vi "Stop Core.vi"(10 "final error code":i32, 11 "WT1600 in":refnum<class "WT1600.lvclass">) -> (3 "WT1600 out":refnum<class "WT1600.lvclass">)   [LabVIEW 2013, in "Universal Power Meter.lvlib" / "WT1600.lvlib" / "WT1600.lvclass"]
doc: "(<B>Filename</B>: Actor Framework.lvlib:Actor.lvclass:Stop Core.vi)\n\nDefines what the actor does before it stops. Use the <B>final error code</B> input to determine whether the actor shut down in response to an error.\n\nBy default, this method does nothing. A descendant class may override it to define behavior, such as shutting down any processes the actor initiated in its override of the Actor Core method."
uses:
  WT1600.lvclass
  Observer Pattern Actor Template/Subject/Subject.lvclass
  <vilib>/ActorFramework/Stop Msg/Stop Msg.lvclass
panel:
  out "error out":errorcluster
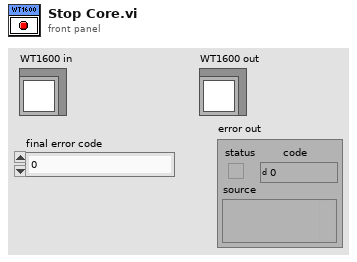
[diagram p1: front panel]
types:
  T1 = cluster{"Card 1":bool, "Card 2":bool, "Card 3":bool, "Card 4":bool, "Card 5":bool, "Card 6":bool}
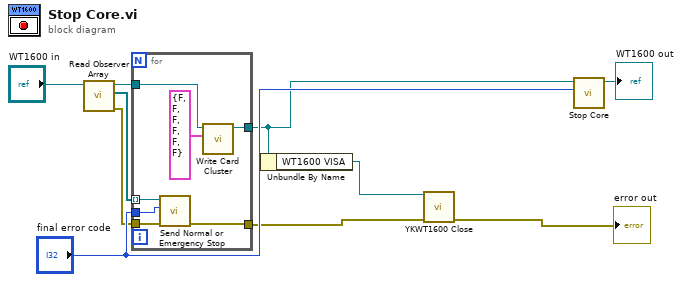
[diagram p0: block diagram]
diagram:
  n1 = call "Read Observer Array.vi"("Subject in"="WT1600 in") -> ("error out"=w5:errorcluster, "Observer Array"=w8:refnum<class "Message Enqueuer.lvclass">[], "Subject out"=w6:refnum<class "WT1600.lvclass">)  [unwired: 8 in]
  n2 = for {
    tunnel: w8 -> [w17] mode=indexing
    tunnel: "final error code" -> [w16]
    tunnel: w6 -> [w15]
    tunnel: [w14] -> w1
    tunnel: w5 -> [w12]
    tunnel: [w11] -> w3
    n3 = call <vilib>:"Send Normal or Emergency Stop.vi"("error in (no error)"=w12, "final error code"=w16, "Message Enqueuer"=w17) -> ("error out"=w11:errorcluster)  [unwired: 8 in]
    n4 = call "Write Card Cluster.vi"("Card Cluster"=T1 {"Card 1"=FALSE, "Card 2"=FALSE, "Card 3"=FALSE, "Card 4"=FALSE, "Card 5"=FALSE, "Card 6"=FALSE}, "WT1600 in"=w15) -> ("WT1600 out"=w14:refnum<class "WT1600.lvclass">)  [unwired: 9 in]
  }
  n5 = Unbundle By Name(w1) -> ("WT1600 VISA"=w4:refnum<visa-resource-name>)
  n6 = call <instrlib>:"YKWT1600 Close.vi"("VISA session"=w4, "error in (no error)"=w3) -> ("error out"=→"error out":errorcluster)  [unwired: 13 in]
  n7 = call-parent "Stop Core.vi"("final error code"="final error code", "Actor in"=w1) -> ("Actor out"=→"WT1600 out":refnum<class "WT1600.lvclass">)  [unwired: 9 in]
